vi "Lab Panel V6.00.vi"() -> ()   [LabVIEW 2017] (continued)
                      frame #2 {
                        # "switch relay off"
                        n3254 = local read "USB OUT 0"() -> (w5922:bool[])
                        n3255 = local read "USB OUT 2"() -> (w5924:bool[])
                        n3256 = local read "USB OUT 1"() -> (w5923:bool[])
                        n3257 = Insert Into Array(array=w5924, index=7, new element=FALSE) -> (w5925:bool[])
                        n3258 = call "sub vi - Drive Relays All v6.vi"("Array #2"=w5925, "Array #1"=w5923, "Array #0"=w5922) -> ()  [unwired: 8 in, 1 out]
                      }
                      frame #3 {
                        # "time delay"
                        n3259 = Wait (ms)(milliseconds to wait=300) -> ()  [unwired: 1 out]
                      }
                      frame #4 {
                        # "read all valid temp circuits"
                        n3260 = local read "LAB01-TP"() -> (w5936:bool)
                        n3261 = local read "LAB03-TP"() -> (w5934:bool)
                        n3262 = local read "LAB02-TP"() -> (w5935:bool)
                        n3263 = local read "LAB04-TP"() -> (w5933:bool)
                        n3264 = local read "LAB05-TP"() -> (w5937:bool)
                        n3265 = call "sub vi - GET ALL TEMP v7.vi"("LA01-EN"=w5936, "LA02-EN"=w5935, "LA03-EN"=w5934, "LA04-EN"=w5933, "LA05-EN"=w5937, "simulate"=w5943, "Gen Cal Value"=w5944) -> ("LOOP TIME"=→"Read Time":dbl, "Fault Counters"=→"Fault Counters":u64[], "error 1"=→"Error Temp":bool, "LA01 TEMP"=w5942:T28, "LA02 TEMP"=w5941:T28, "LA04 TEMP"=w5939:T28, "LA03 TEMP"=w5940:T28, "Errors"=→"TempErrors":bool[], "LA05 TEMP"=w5938:T28)  [unwired: 3 in, 1 out]
                        n3266 = local write "LAB01 TEMP"(w5942) -> ()
                        n3267 = local write "LAB02 TEMP"(w5941) -> ()
                        n3268 = local write "LAB03 TEMP"(w5940) -> ()
                        n3269 = local write "LAB04 TEMP"(w5939) -> ()
                        n3270 = local write "LAB05 TEMP"(w5938) -> ()
                      }
                    }
                  }
                }
              }
              frame #2 {
                n3271 = case shown="True" w5945 {
                  tunnel: w5958 -> [_ w5971]
                  tunnel: w5957 -> [_ w5970]
                  tunnel: w5956 -> [_ w5969]
                  tunnel: w5955 -> [_ w5968]
                  tunnel: w5954 -> [_ w5967]
                  tunnel: w5953 -> [_ w5966]
                  tunnel: w5952 -> [_ w5965]
                  tunnel: w5951 -> [_ w5964]
                  tunnel: w5950 -> [_ w5963]
                  tunnel: w5949 -> [_ w5962]
                  tunnel: w5948 -> [_ w5961]
                  tunnel: w5947 -> [_ w5960]
                  tunnel: w5946 -> [_ w5959]
                  frame False {
                  }
                  frame True {
                    n3272 = stacked-sequence {
                      tunnel: w5971 -> [_ w5984 w6029 w6074 w6119 w6164 _]
                      tunnel: w5970 -> [_ w5983 w6028 w6073 w6118 w6163 _]
                      tunnel: w5969 -> [_ w5973 _ _ _ _ _]
                      tunnel: w5968 -> [_ w5978 w6027 w6072 w6117 w6162 _]
                      tunnel: w5967 -> [_ w5972 _ _ _ _ _]
                      tunnel: w5966 -> [_ _ w6018 _ _ _ _]
                      tunnel: w5965 -> [_ _ w6017 _ _ _ _]
                      tunnel: w5964 -> [_ _ _ w6063 _ _ _]
                      tunnel: w5963 -> [_ _ _ w6062 _ _ _]
                      tunnel: w5962 -> [_ _ _ _ w6108 _ _]
                      tunnel: w5961 -> [_ _ _ _ w6107 _ _]
                      tunnel: w5960 -> [_ _ _ _ _ w6153 _]
                      tunnel: w5959 -> [_ _ _ _ _ w6152 _]
                      frame #0 {
                      }
                      frame #1 {
                        n3273 = case shown="False" w5984 {
                          tunnel: [w6015 w6016] -> w6000
                          tunnel: w5983 -> [_ w6016]
                          frame False {
                            n3274 = local read "CAL LAB01"() -> (w6015:T15)
                          }
                          frame True {
                          }
                        }
                        n3275 = local read "TEMP LA01"() -> (w5991:T10)
                        n3276 = local read "LAB01 TEMP"() -> (w5990:T13)
                        n3277 = call "sub vi - temperature delay v4.vi"("2-run"=w5972, "1-run"=w5973, "temp values IN"=w5991, "temp signals"=w5990) -> ("T2-N"=w5986:dbl, "T2-L"=w5987:dbl, "T1-N"=w5988:dbl, "T1-L"=w5989:dbl, "temp values OUT"=w5985:T48)  [unwired: 3 in]
                        n3278 = Unbundle By Name(w6000) -> ("1 (TL) cal"=w5995:dbl, "1 (TN) cal"=w5994:dbl, "2 (TL) cal"=w5993:dbl, "2 (TN) cal"=w5992:dbl)  [unwired: 6 out]
                        n3279 = local write "TEMP LA01"(w5985) -> ()
                        n3280 = Multiply(x=w5989, y=w5995) -> (x*y=w5982:dbl)
                        n3281 = Multiply(x=w5988, y=w5994) -> (x*y=w5980:dbl)
                        n3282 = Multiply(x=w5987, y=w5993) -> (x*y=w5977:dbl)
                        n3283 = Multiply(x=w5986, y=w5992) -> (x*y=w5976:dbl)
                        n3284 = case shown="True" w5973 {
                          tunnel: w5982 -> [w6009 w6014]
                          tunnel: w5978 -> [_ w6012]
                          tunnel: [w6009 w6013] -> w5981
                          tunnel: w5980 -> [w6008 w6011]
                          tunnel: [w6008 w6010] -> w5979
                          frame False {
                          }
                          frame True {
                            n3285 = Multiply(x=w6012, y=w6011) -> (x*y=w6010:dbl)
                            n3286 = Multiply(x=w6012, y=w6014) -> (x*y=w6013:dbl)
                          }
                        }
                        n3287 = case shown="True" w5972 {
                          tunnel: w5977 -> [w6002 w6007]
                          tunnel: w5978 -> [_ w6005]
                          tunnel: [w6002 w6006] -> w5975
                          tunnel: w5976 -> [w6001 w6004]
                          tunnel: [w6001 w6003] -> w5974
                          frame False {
                          }
                          frame True {
                            n3288 = Multiply(x=w6005, y=w6004) -> (x*y=w6003:dbl)
                            n3289 = Multiply(x=w6005, y=w6007) -> (x*y=w6006:dbl)
                          }
                        }
                        n3290 = local read "SIG LAB01-2"() -> (w5997:T2)
                        n3291 = local read "SIG LAB01-1"() -> (w5999:T2)
                        n3292 = Bundle By Name(cluster=w5999, "Tmp Live"=w5981, "Tmp Neut"=w5979) -> (w5998:T2)
                        n3293 = Bundle By Name(cluster=w5997, "Tmp Live"=w5975, "Tmp Neut"=w5974) -> (w5996:T2)
                        n3294 = local write "SIG LAB01-1"(w5998) -> ()
                        n3295 = local write "SIG LAB01-2"(w5996) -> ()
                      }
                      frame #2 {
                        n3296 = case shown="True" w6029 {
                          tunnel: [w6060 w6061] -> w6045
                          tunnel: w6028 -> [_ w6061]
                          frame False {
                            n3297 = local read "CAL LAB02"() -> (w6060:T16)
                          }
                          frame True {
                          }
                        }
                        n3298 = local read "LAB02 TEMP"() -> (w6036:T13)
                        n3299 = local read "TEMP LA02"() -> (w6035:T10)
                        n3300 = call "sub vi - temperature delay v4.vi"("2-run"=w6017, "1-run"=w6018, "temp values IN"=w6035, "temp signals"=w6036) -> ("T2-N"=w6030:dbl, "T2-L"=w6031:dbl, "T1-N"=w6032:dbl, "T1-L"=w6033:dbl, "temp values OUT"=w6034:T48)  [unwired: 3 in]
                        n3301 = Unbundle By Name(w6045) -> ("1 (TL) cal"=w6040:dbl, "1 (TN) cal"=w6039:dbl, "2 (TL) cal"=w6038:dbl, "2 (TN) cal"=w6037:dbl)  [unwired: 6 out]
                        n3302 = local write "TEMP LA02"(w6034) -> ()
                        n3303 = Multiply(x=w6033, y=w6040) -> (x*y=w6026:dbl)
                        n3304 = Multiply(x=w6032, y=w6039) -> (x*y=w6025:dbl)
                        n3305 = Multiply(x=w6031, y=w6038) -> (x*y=w6022:dbl)
                        n3306 = Multiply(x=w6030, y=w6037) -> (x*y=w6021:dbl)
                        n3307 = case shown="True" w6018 {
                          tunnel: w6026 -> [w6054 w6059]
                          tunnel: w6027 -> [_ w6057]
                          tunnel: [w6054 w6058] -> w6024
                          tunnel: w6025 -> [w6053 w6056]
                          tunnel: [w6053 w6055] -> w6023
                          frame False {
                          }
                          frame True {
                            n3308 = Multiply(x=w6057, y=w6056) -> (x*y=w6055:dbl)
                            n3309 = Multiply(x=w6057, y=w6059) -> (x*y=w6058:dbl)
                          }
                        }
                        n3310 = case shown="True" w6017 {
                          tunnel: w6022 -> [w6047 w6052]
                          tunnel: w6027 -> [_ w6050]
                          tunnel: [w6047 w6051] -> w6020
                          tunnel: w6021 -> [w6046 w6049]
                          tunnel: [w6046 w6048] -> w6019
                          frame False {
                          }
                          frame True {
                            n3311 = Multiply(x=w6050, y=w6049) -> (x*y=w6048:dbl)
                            n3312 = Multiply(x=w6050, y=w6052) -> (x*y=w6051:dbl)
                          }
                        }
                        n3313 = local read "SIG LAB02-2"() -> (w6042:T2)
                        n3314 = local read "SIG LAB02-1"() -> (w6044:T2)
                        n3315 = Bundle By Name(cluster=w6042, "Tmp Live"=w6020, "Tmp Neut"=w6019) -> (w6041:T2)
                        n3316 = Bundle By Name(cluster=w6044, "Tmp Live"=w6024, "Tmp Neut"=w6023) -> (w6043:T2)
                        n3317 = local write "SIG LAB02-1"(w6043) -> ()
                        n3318 = local write "SIG LAB02-2"(w6041) -> ()
                      }
                      frame #3 {
                        n3319 = case shown="False" w6074 {
                          tunnel: [w6105 w6106] -> w6090
                          tunnel: w6073 -> [_ w6106]
                          frame False {
                            n3320 = local read "CAL LAB03"() -> (w6105:T15)
                          }
                          frame True {
                          }
                        }
                        n3321 = local read "TEMP LA03"() -> (w6080:T10)
                        n3322 = local read "LAB03 TEMP"() -> (w6081:T13)
                        n3323 = call "sub vi - temperature delay v4.vi"("2-run"=w6062, "1-run"=w6063, "temp values IN"=w6080, "temp signals"=w6081) -> ("T2-N"=w6075:dbl, "T2-L"=w6076:dbl, "T1-N"=w6077:dbl, "T1-L"=w6078:dbl, "temp values OUT"=w6079:T48)  [unwired: 3 in]
                        n3324 = Unbundle By Name(w6090) -> ("1 (TL) cal"=w6085:dbl, "1 (TN) cal"=w6084:dbl, "2 (TL) cal"=w6083:dbl, "2 (TN) cal"=w6082:dbl)  [unwired: 6 out]
                        n3325 = local write "TEMP LA03"(w6079) -> ()
                        n3326 = Multiply(x=w6078, y=w6085) -> (x*y=w6071:dbl)
                        n3327 = Multiply(x=w6077, y=w6084) -> (x*y=w6070:dbl)
                        n3328 = Multiply(x=w6076, y=w6083) -> (x*y=w6067:dbl)
                        n3329 = Multiply(x=w6075, y=w6082) -> (x*y=w6066:dbl)
                        n3330 = case shown="True" w6062 {
                          tunnel: w6067 -> [w6092 w6097]
                          tunnel: w6072 -> [_ w6095]
                          tunnel: [w6092 w6096] -> w6065
                          tunnel: w6066 -> [w6091 w6094]
                          tunnel: [w6091 w6093] -> w6064
                          frame False {
                          }
                          frame True {
                            n3331 = Multiply(x=w6095, y=w6094) -> (x*y=w6093:dbl)
                            n3332 = Multiply(x=w6095, y=w6097) -> (x*y=w6096:dbl)
                          }
                        }
                        n3333 = case shown="True" w6063 {
                          tunnel: w6071 -> [w6099 w6104]
                          tunnel: w6072 -> [_ w6102]
                          tunnel: [w6099 w6103] -> w6069
                          tunnel: w6070 -> [w6098 w6101]
                          tunnel: [w6098 w6100] -> w6068
                          frame False {
                          }
                          frame True {
                            n3334 = Multiply(x=w6102, y=w6101) -> (x*y=w6100:dbl)
                            n3335 = Multiply(x=w6102, y=w6104) -> (x*y=w6103:dbl)
                          }
                        }
                        n3336 = local read "SIG LAB03-2"() -> (w6087:T2)
                        n3337 = local read "SIG LAB03-1"() -> (w6089:T2)
                        n3338 = Bundle By Name(cluster=w6087, "Tmp Live"=w6065, "Tmp Neut"=w6064) -> (w6086:T2)
                        n3339 = Bundle By Name(cluster=w6089, "Tmp Live"=w6069, "Tmp Neut"=w6068) -> (w6088:T2)
                        n3340 = local write "SIG LAB03-2"(w6086) -> ()
                        n3341 = local write "SIG LAB03-1"(w6088) -> ()
                      }
                      frame #4 {
                        n3342 = case shown="False" w6119 {
                          tunnel: [w6150 w6151] -> w6135
                          tunnel: w6118 -> [_ w6151]
                          frame False {
                            n3343 = local read "CAL LAB04"() -> (w6150:T15)
                          }
                          frame True {
                          }
                        }
                        n3344 = local read "LAB04 TEMP"() -> (w6125:T13)
                        n3345 = local read "TEMP LA04"() -> (w6126:T10)
                        n3346 = call "sub vi - temperature delay v4.vi"("2-run"=w6107, "1-run"=w6108, "temp values IN"=w6126, "temp signals"=w6125) -> ("T2-N"=w6120:dbl, "T2-L"=w6121:dbl, "T1-N"=w6122:dbl, "T1-L"=w6123:dbl, "temp values OUT"=w6124:T48)  [unwired: 3 in]
                        n3347 = Unbundle By Name(w6135) -> ("1 (TL) cal"=w6130:dbl, "1 (TN) cal"=w6129:dbl, "2 (TL) cal"=w6128:dbl, "2 (TN) cal"=w6127:dbl)  [unwired: 6 out]
                        n3348 = local write "TEMP LA04"(w6124) -> ()
                        n3349 = Multiply(x=w6123, y=w6130) -> (x*y=w6116:dbl)
                        n3350 = Multiply(x=w6122, y=w6129) -> (x*y=w6115:dbl)
                        n3351 = Multiply(x=w6121, y=w6128) -> (x*y=w6112:dbl)
                        n3352 = Multiply(x=w6120, y=w6127) -> (x*y=w6111:dbl)
                        n3353 = case shown="True" w6107 {
                          tunnel: w6112 -> [w6137 w6142]
                          tunnel: w6117 -> [_ w6140]
                          tunnel: [w6137 w6141] -> w6110
                          tunnel: w6111 -> [w6136 w6139]
                          tunnel: [w6136 w6138] -> w6109
                          frame False {
                          }
                          frame True {
                            n3354 = Multiply(x=w6140, y=w6139) -> (x*y=w6138:dbl)
                            n3355 = Multiply(x=w6140, y=w6142) -> (x*y=w6141:dbl)
                          }
                        }
                        n3356 = case shown="True" w6108 {
                          tunnel: w6116 -> [w6144 w6149]
                          tunnel: w6117 -> [_ w6147]
                          tunnel: [w6144 w6148] -> w6114
                          tunnel: w6115 -> [w6143 w6146]
                          tunnel: [w6143 w6145] -> w6113
                          frame False {
                          }
                          frame True {
                            n3357 = Multiply(x=w6147, y=w6146) -> (x*y=w6145:dbl)
                            n3358 = Multiply(x=w6147, y=w6149) -> (x*y=w6148:dbl)
                          }
                        }
                        n3359 = local read "SIG LAB04-2"() -> (w6132:T2)
                        n3360 = local read "SIG LAB04-1"() -> (w6134:T2)
                        n3361 = Bundle By Name(cluster=w6132, "Tmp Live"=w6110, "Tmp Neut"=w6109) -> (w6131:T2)
                        n3362 = Bundle By Name(cluster=w6134, "Tmp Live"=w6114, "Tmp Neut"=w6113) -> (w6133:T2)
                        n3363 = local write "SIG LAB04-2"(w6131) -> ()
                        n3364 = local write "SIG LAB04-1"(w6133) -> ()
                      }
                      frame #5 {
                        n3365 = case shown="False" w6164 {
                          tunnel: [w6195 w6196] -> w6180
                          tunnel: w6163 -> [_ w6196]
                          frame False {
                            n3366 = local read "CAL LAB05"() -> (w6195:T15)
                          }
                          frame True {
                          }
                        }
                        n3367 = local read "LAB05 TEMP"() -> (w6170:T13)
                        n3368 = local read "TEMP LA05"() -> (w6171:T10)
                        n3369 = call "sub vi - temperature delay v4.vi"("2-run"=w6152, "1-run"=w6153, "temp values IN"=w6171, "temp signals"=w6170) -> ("T2-N"=w6166:dbl, "T2-L"=w6167:dbl, "T1-N"=w6168:dbl, "T1-L"=w6169:dbl, "temp values OUT"=w6165:T48)  [unwired: 3 in]
                        n3370 = local write "TEMP LA05"(w6165) -> ()
                        n3371 = Unbundle By Name(w6180) -> ("1 (TL) cal"=w6172:dbl, "1 (TN) cal"=w6175:dbl, "2 (TL) cal"=w6174:dbl, "2 (TN) cal"=w6173:dbl)  [unwired: 6 out]
                        n3372 = Multiply(x=w6169, y=w6172) -> (x*y=w6161:dbl)
                        n3373 = Multiply(x=w6168, y=w6175) -> (x*y=w6160:dbl)
                        n3374 = Multiply(x=w6167, y=w6174) -> (x*y=w6157:dbl)
                        n3375 = Multiply(x=w6166, y=w6173) -> (x*y=w6156:dbl)
                        n3376 = case shown="True" w6152 {
                          tunnel: w6157 -> [w6182 w6187]
                          tunnel: w6162 -> [_ w6185]
                          tunnel: [w6182 w6186] -> w6155
                          tunnel: w6156 -> [w6181 w6184]
                          tunnel: [w6181 w6183] -> w6154
                          frame False {
                          }
                          frame True {
                            n3377 = Multiply(x=w6185, y=w6184) -> (x*y=w6183:dbl)
                            n3378 = Multiply(x=w6185, y=w6187) -> (x*y=w6186:dbl)
                          }
                        }
                        n3379 = case shown="True" w6153 {
                          tunnel: w6161 -> [w6189 w6194]
                          tunnel: w6162 -> [_ w6192]
                          tunnel: [w6189 w6193] -> w6159
                          tunnel: w6160 -> [w6188 w6191]
                          tunnel: [w6188 w6190] -> w6158
                          frame False {
                          }
                          frame True {
                            n3380 = Multiply(x=w6192, y=w6191) -> (x*y=w6190:dbl)
                            n3381 = Multiply(x=w6192, y=w6194) -> (x*y=w6193:dbl)
                          }
                        }
                        n3382 = local read "SIG LAB05-1"() -> (w6179:T2)
                        n3383 = Bundle By Name(cluster=w6179, "Tmp Live"=w6159, "Tmp Neut"=w6158) -> (w6178:T2)
                        n3384 = local read "SIG LAB05-2"() -> (w6177:T2)
                        n3385 = Bundle By Name(cluster=w6177, "Tmp Live"=w6155, "Tmp Neut"=w6154) -> (w6176:T2)
                        n3386 = local write "SIG LAB05-1"(w6178) -> ()
                        n3387 = local write "SIG LAB05-2"(w6176) -> ()
                      }
                      frame #6 {
                        w6297 = 150.0
                        # "check for thermocouple error, output >150 deg??"
                        n3388 = local read "SIG LAB01-2"() -> (w6306:T2)
                        n3389 = local read "SIG LAB01-1"() -> (w6307:T2)
                        n3390 = local read "SIG LAB04-1"() -> (w6300:T2)
                        n3391 = local read "SIG LAB04-2"() -> (w6301:T2)
                        n3392 = Unbundle By Name(w6307) -> ("Tmp Live"=w6235:dbl, "Tmp Neut"=w6233:dbl)
                        n3393 = Unbundle(w6301) -> ("Tmp Live"=w6211:dbl, "Tmp Neut"=w6210:dbl)  [unwired: 3 out]
                        n3394 = Unbundle(w6306) -> ("Tmp Live"=w6232:dbl, "Tmp Neut"=w6230:dbl)  [unwired: 3 out]
                        n3395 = Unbundle(w6300) -> ("Tmp Live"=w6212:dbl, "Tmp Neut"=w6205:dbl)  [unwired: 3 out]
                        n3396 = Absolute Value(x=w6212) -> (abs(x)=w6206:dbl)
                        n3397 = Absolute Value(x=w6205) -> (abs(x)=w6207:dbl)
                        n3398 = Absolute Value(x=w6211) -> (abs(x)=w6209:dbl)
                        n3399 = Absolute Value(x=w6210) -> (abs(x)=w6208:dbl)
                        n3400 = Absolute Value(x=w6232) -> (abs(x)=w6231:dbl)
                        n3401 = Absolute Value(x=w6230) -> (abs(x)=w6229:dbl)
                        n3402 = Absolute Value(x=w6233) -> (abs(x)=w6234:dbl)
                        n3403 = Absolute Value(x=w6235) -> (abs(x)=w6236:dbl)
                        n3404 = Greater?(x=w6208, y=w6297) -> (0:w6273:bool)
                        "LA04-2 (TN)" <- w6273
                        n3405 = Greater?(x=w6229, y=w6297) -> (0:w6285:bool)
                        "LA01-2 (TN)" <- w6285
                        n3406 = Greater?(x=w6209, y=w6297) -> (0:w6274:bool)
                        "LA04-2 (TL)" <- w6274
                        n3407 = Greater?(x=w6231, y=w6297) -> (0:w6286:bool)
                        "LA01-2 (TL)" <- w6286
                        n3408 = Greater?(x=w6207, y=w6297) -> (0:w6275:bool)
                        "LA04-1 (TN)" <- w6275
                        n3409 = Greater?(x=w6234, y=w6297) -> (0:w6296:bool)
                        "LA01-1 (TN)" <- w6296
                        n3410 = Greater?(x=w6206, y=w6297) -> (0:w6276:bool)
                        "LA04-1 (TL)" <- w6276
                        n3411 = Greater?(x=w6236, y=w6297) -> (0:w6295:bool)
                        "LA01-1 (TL)" <- w6295
                        n3412 = Or(x=w6296, y=w6295) -> (x .or. y?=w6294:bool)
                        n3413 = Or(x=w6273, y=w6274) -> (x .or. y?=w6284:bool)
                        n3414 = Or(x=w6286, y=w6285) -> (x .or. y?=w6290:bool)
                        n3415 = Or(x=w6275, y=w6276) -> (x .or. y?=w6280:bool)
                        n3416 = Select(t=u32 16711680, s=w6294, f=u32 13816530) -> (s? t:f=w6291:u32)
                        n3417 = Select(t=u32 16711680, s=w6284, f=u32 13816530) -> (s? t:f=w6281:u32)
                        n3418 = Select(t=u32 16711680, s=w6290, f=u32 13816530) -> (s? t:f=w6287:u32)
                        n3419 = Select(t=u32 16711680, s=w6280, f=u32 13816530) -> (s? t:f=w6277:u32)
                        n3420 = property on="SIG LAB01-1" class="Clust (strict)"("Color"=w6291) -> ()  [unwired: 2 in, 2 out]
                        n3421 = property on="SIG LAB01-2" class="Clust (strict)"("Color"=w6287) -> ()  [unwired: 2 in, 2 out]
                        n3422 = property on="SIG LAB04-2" class="Clust (strict)"("Color"=w6281) -> ()  [unwired: 2 in, 2 out]
                        n3423 = property on="SIG LAB04-1" class="Clust (strict)"("Color"=w6277) -> ()  [unwired: 2 in, 2 out]
                        n3424 = local read "SIG LAB02-1"() -> (w6304:T2)
                        n3425 = local read "SIG LAB02-2"() -> (w6305:T2)
                        n3426 = local read "SIG LAB05-2"() -> (w6298:T2)
                        n3427 = local read "SIG LAB05-1"() -> (w6299:T2)
                        n3428 = Unbundle(w6305) -> ("Tmp Live"=w6224:dbl, "Tmp Neut"=w6222:dbl)  [unwired: 3 out]
                        n3429 = Unbundle(w6304) -> ("Tmp Live"=w6228:dbl, "Tmp Neut"=w6227:dbl)  [unwired: 3 out]
                        n3430 = Unbundle(w6298) -> ("Tmp Live"=w6200:dbl, "Tmp Neut"=w6198:dbl)  [unwired: 3 out]
                        n3431 = Unbundle(w6299) -> ("Tmp Live"=w6204:dbl, "Tmp Neut"=w6202:dbl)  [unwired: 3 out]
                        n3432 = Absolute Value(x=w6224) -> (abs(x)=w6223:dbl)
                        n3433 = Absolute Value(x=w6222) -> (abs(x)=w6221:dbl)
                        n3434 = Absolute Value(x=w6227) -> (abs(x)=w6225:dbl)
                        n3435 = Absolute Value(x=w6228) -> (abs(x)=w6226:dbl)
                        n3436 = Absolute Value(x=w6200) -> (abs(x)=w6199:dbl)
                        n3437 = Absolute Value(x=w6198) -> (abs(x)=w6197:dbl)
                        n3438 = Absolute Value(x=w6204) -> (abs(x)=w6203:dbl)
                        n3439 = Absolute Value(x=w6202) -> (abs(x)=w6201:dbl)
                        n3440 = Greater?(x=w6221, y=w6297) -> (0:w6249:bool)
                        "LA02-2 (TN)" <- w6249
                        n3441 = Greater?(x=w6223, y=w6297) -> (0:w6250:bool)
                        "LA02-2 (TL)" <- w6250
                        n3442 = Greater?(x=w6225, y=w6297) -> (0:w6252:bool)
                        "LA02-1 (TN)" <- w6252
                        n3443 = Greater?(x=w6226, y=w6297) -> (0:w6251:bool)
                        "LA02-1 (TL)" <- w6251
                        n3444 = Greater?(x=w6197, y=w6297) -> (0:w6261:bool)
                        "LA05-2 (TN)" <- w6261
                        n3445 = Greater?(x=w6199, y=w6297) -> (0:w6262:bool)
                        "LA05-2 (TL)" <- w6262
                        n3446 = Greater?(x=w6201, y=w6297) -> (0:w6263:bool)
                        "LA05-1 (TN)" <- w6263
                        n3447 = Greater?(x=w6203, y=w6297) -> (0:w6264:bool)
                        "LA05-1 (TL)" <- w6264
                        n3448 = Or(x=w6252, y=w6251) -> (x .or. y?=w6260:bool)
                        n3449 = Or(x=w6250, y=w6249) -> (x .or. y?=w6256:bool)
                        n3450 = Or(x=w6264, y=w6263) -> (x .or. y?=w6272:bool)
                        n3451 = Or(x=w6262, y=w6261) -> (x .or. y?=w6268:bool)
                        n3452 = Select(t=u32 16711680, s=w6260, f=u32 13816530) -> (s? t:f=w6257:u32)
                        n3453 = Select(t=u32 16711680, s=w6256, f=u32 13816530) -> (s? t:f=w6253:u32)
                        n3454 = Select(t=u32 16711680, s=w6272, f=u32 13816530) -> (s? t:f=w6269:u32)
                        n3455 = local read "SIG LAB03-1"() -> (w6302:T2)
                        n3456 = Select(t=u32 16711680, s=w6268, f=u32 13816530) -> (s? t:f=w6265:u32)
                        n3457 = property on="SIG LAB02-1" class="Clust (strict)"("Color"=w6257) -> ()  [unwired: 2 in, 2 out]
                        n3458 = property on="SIG LAB02-2" class="Clust (strict)"("Color"=w6253) -> ()  [unwired: 2 in, 2 out]
                        n3459 = local read "SIG LAB03-2"() -> (w6303:T2)
                        n3460 = property on="SIG LAB05-1" class="Clust (strict)"("Color"=w6269) -> ()  [unwired: 2 in, 2 out]
                        n3461 = property on="SIG LAB05-2" class="Clust (strict)"("Color"=w6265) -> ()  [unwired: 2 in, 2 out]
                        n3462 = Unbundle(w6303) -> ("Tmp Live"=w6216:dbl, "Tmp Neut"=w6214:dbl)  [unwired: 3 out]
                        n3463 = Unbundle(w6302) -> ("Tmp Live"=w6220:dbl, "Tmp Neut"=w6218:dbl)  [unwired: 3 out]
                        n3464 = Absolute Value(x=w6216) -> (abs(x)=w6215:dbl)
                        n3465 = Absolute Value(x=w6214) -> (abs(x)=w6213:dbl)
                        n3466 = Absolute Value(x=w6220) -> (abs(x)=w6219:dbl)
                        n3467 = Absolute Value(x=w6218) -> (abs(x)=w6217:dbl)
                        n3468 = Greater?(x=w6213, y=w6297) -> (0:w6237:bool)
                        "LA03-2 (TN)" <- w6237
                        n3469 = Greater?(x=w6215, y=w6297) -> (0:w6238:bool)
                        "LA03-2 (TL)" <- w6238
                        n3470 = Greater?(x=w6217, y=w6297) -> (0:w6240:bool)
                        "LA03-1 (TN)" <- w6240
                        n3471 = Greater?(x=w6219, y=w6297) -> (0:w6239:bool)
                        "LA03-1 (TL)" <- w6239
                        n3472 = Or(x=w6240, y=w6239) -> (x .or. y?=w6248:bool)
                        n3473 = Or(x=w6238, y=w6237) -> (x .or. y?=w6244:bool)
                        n3474 = Select(t=u32 16711680, s=w6248, f=u32 13816530) -> (s? t:f=w6245:u32)
                        n3475 = Select(t=u32 16711680, s=w6244, f=u32 13816530) -> (s? t:f=w6241:u32)
                        n3476 = property on="SIG LAB03-1" class="Clust (strict)"("Color"=w6245) -> ()  [unwired: 2 in, 2 out]
                        n3477 = property on="SIG LAB03-2" class="Clust (strict)"("Color"=w6241) -> ()  [unwired: 2 in, 2 out]
                      }
                    }
                  }
                }
              }
            }
          }
          frame #22 {
            # "SAVE ON AMPS VALUES FOR REPORT FILE"
            # "write data to display panel"
            n3478 = global write "Global display 1.vi" "TEST 5-2"(w6343) -> ()
            n3479 = global write "Global display 1.vi" "TEST 4-2"(w6345) -> ()
            n3480 = global write "Global display 1.vi" "TEST 1-2"(w6351) -> ()
            n3481 = global write "Global display 1.vi" "TEST 3-1"(w6348) -> ()
            n3482 = global write "Global display 1.vi" "TEST 5-1"(w6344) -> ()
            n3483 = global write "Global display 1.vi" "TEST 1-1"(w6352) -> ()
            n3484 = global write "Global display 1.vi" "TEST 3-2"(w6347) -> ()
            n3485 = global write "Global display 1.vi" "TEST 4-1"(w6346) -> ()
            n3486 = global write "Global display 1.vi" "TEST 2-2"(w6349) -> ()
            n3487 = global write "Global display 1.vi" "TEST 2-1"(w6350) -> ()
            n3488 = global read "Global display 3.vi" "log 1-1"() -> (→"LOG LAB01-1":string)
            n3489 = global read "Global display 3.vi" "log 3-1"() -> (→"LOG LAB03-1":string)
            n3490 = global read "Global display 3.vi" "log 1-2"() -> (→"LOG LAB01-2":string)
            n3491 = property on="Tab Control 2" class="TabCtl (strict)"() -> ("Pages"=w6342:refnum<vi>[])  [unwired: 2 in, 2 out]
            n3492 = global read "Global display 3.vi" "log 2-1"() -> (→"LOG LAB02-1":string)
            n3493 = global read "Global display 3.vi" "log 2-2"() -> (→"LOG LAB02-2":string)
            n3494 = global read "Global display 3.vi" "log 4-2"() -> (→"LOG LAB04-2":string)
            n3495 = global read "Global display 3.vi" "log 5-2"() -> (→"LOG LAB05-2":string)
            n3496 = global read "Global display 3.vi" "log 5-1"() -> (→"LOG LAB05-1":string)
            n3497 = global read "Global display 3.vi" "log 4-1"() -> (→"LOG LAB04-1":string)
            n3498 = global read "Global display 3.vi" "log 3-2"() -> (→"LOG LAB03-2":string)
            n3499 = Index Array(array=w6342, index=8) -> (element=w6340:refnum<vi>)
            n3500 = property class="Page"(reference=w6340) -> ("PageVis"=w6339:bool)  [unwired: 1 in, 2 out]
            n3501 = local read "DISP LAB03-1"() -> (w6378:T4)
            n3502 = local read "DISP LAB04-2"() -> (w6375:T4)
            n3503 = local read "DISP LAB05-1"() -> (w6374:T4)
            n3504 = local read "DISP LAB01-2"() -> (w6381:T4)
            n3505 = local read "DISP LAB02-1"() -> (w6380:T4)
            n3506 = local read "DISP LAB02-2"() -> (w6379:T4)
            n3507 = local read "DISP LAB04-1"() -> (w6376:T4)
            n3508 = local read "DISP LAB05-2"() -> (w6373:T4)
            n3509 = local read "DISP LAB01-1"() -> (w6382:T4)
            n3510 = local read "DISP LAB03-2"() -> (w6377:T4)
            n3511 = global write "Global display 3.vi" "admin"(w6339) -> ()
            n3512 = local read "O/I  LAB05-2"() -> (w6393:bool)
            n3513 = local read "O/I  LAB05-1"() -> (w6394:bool)
            n3514 = local read "O/I  LAB03-2"() -> (w6397:bool)
            n3515 = local read "O/I  LAB04-2"() -> (w6395:bool)
            n3516 = local read "O/I  LAB04-1"() -> (w6396:bool)
            n3517 = local read "O/I  LAB03-1"() -> (w6398:bool)
            n3518 = local read "O/I  LAB01-2"() -> (w6401:bool)
            n3519 = local read "O/I  LAB01-1"() -> (w6402:bool)
            n3520 = local read "O/I  LAB02-1"() -> (w6400:bool)
            n3521 = local read "O/I  LAB02-2"() -> (w6399:bool)
            n3522 = global write "Global display 1.vi" "5-2 O/F"(w6393) -> ()
            n3523 = global write "Global display 1.vi" "5-1 O/F"(w6394) -> ()
            n3524 = global write "Global display 1.vi" "4-1 O/F"(w6396) -> ()
            n3525 = global write "Global display 1.vi" "4-2 O/F"(w6395) -> ()
            n3526 = global write "Global display 2.vi" "DISP LAB02-1"(w6380) -> ()
            n3527 = global write "Global display 2.vi" "DISP LAB02-2"(w6379) -> ()
            n3528 = global write "Global display 2.vi" "DISP LAB05-1"(w6374) -> ()
            n3529 = global write "Global display 2.vi" "DISP LAB05-2"(w6373) -> ()
            n3530 = global write "Global display 1.vi" "3-2 O/F"(w6397) -> ()
            n3531 = global write "Global display 2.vi" "DISP LAB01-2"(w6381) -> ()
            n3532 = global write "Global display 2.vi" "DISP LAB04-2"(w6375) -> ()
            n3533 = global write "Global display 2.vi" "DISP LAB01-1"(w6382) -> ()
            n3534 = global write "Global display 2.vi" "DISP LAB03-1"(w6378) -> ()
            n3535 = global write "Global display 1.vi" "3-1 O/F"(w6398) -> ()
            n3536 = global write "Global display 2.vi" "DISP LAB04-1"(w6376) -> ()
            n3537 = global write "Global display 1.vi" "2-2 O/F"(w6399) -> ()
            n3538 = global write "Global display 2.vi" "DISP LAB03-2"(w6377) -> ()
            n3539 = global write "Global display 1.vi" "2-1 O/F"(w6400) -> ()
            n3540 = global write "Global display 1.vi" "1-2 O/F"(w6401) -> ()
            n3541 = global write "Global display 1.vi" "1-1 O/F"(w6402) -> ()
            n3542 = local read "run lab05-2"() -> (w6383:bool)
            n3543 = local read "run lab04-1"() -> (w6386:bool)
            n3544 = local read "run lab04-2"() -> (w6385:bool)
            n3545 = local read "run lab05-1"() -> (w6384:bool)
            n3546 = local read "TEMP START LAB02-2"() -> (w6325:cluster{"TL":dbl, "TN":dbl})
            n3547 = local read "TEMP START LAB01-2"() -> (w6327:cluster{"TL":dbl, "TN":dbl})
            n3548 = local read "TEMP START LAB02-1"() -> (w6326:cluster{"TL":dbl, "TN":dbl})
            n3549 = local read "TEMP START LAB04-1"() -> (w6322:cluster{"TL":dbl, "TN":dbl})
            n3550 = local read "TEMP START LAB04-2"() -> (w6321:cluster{"TL":dbl, "TN":dbl})
            n3551 = local read "run lab03-2"() -> (w6387:bool)
            n3552 = local read "TEMP START LAB01-1"() -> (w6328:cluster{"TL":dbl, "TN":dbl})
            n3553 = local read "TEMP START LAB05-2"() -> (w6319:cluster{"TL":dbl, "TN":dbl})
            n3554 = local read "TEMP START LAB05-1"() -> (w6320:cluster{"TL":dbl, "TN":dbl})
            n3555 = local read "run lab02-1"() -> (w6390:bool)
            n3556 = local read "run lab03-1"() -> (w6388:bool)
            n3557 = local read "TEMP START LAB03-2"() -> (w6323:cluster{"TL":dbl, "TN":dbl})
            n3558 = local read "run lab01-2"() -> (w6391:bool)
            n3559 = local read "run lab02-2"() -> (w6389:bool)
            n3560 = local read "TEMP START LAB03-1"() -> (w6324:cluster{"TL":dbl, "TN":dbl})
            n3561 = local read "run lab01-1"() -> (w6392:bool)
            n3562 = global write "Global display 1.vi" "5-2 R/S"(w6383) -> ()
            n3563 = global write "Global display 1.vi" "5-1 R/S"(w6384) -> ()
            n3564 = global write "Global display 1.vi" "4-2 R/S"(w6385) -> ()
            n3565 = global write "Global display 1.vi" "4-1 R/S"(w6386) -> ()
            n3566 = global write "Global display 1.vi" "3-2 R/S"(w6387) -> ()
            n3567 = global write "Global display 1.vi" "1-2 R/S"(w6391) -> ()
            n3568 = global write "Global display 1.vi" "2-1 R/S"(w6390) -> ()
            n3569 = global write "Global display 1.vi" "3-1 R/S"(w6388) -> ()
            n3570 = global write "Global display 1.vi" "2-2 R/S"(w6389) -> ()
            n3571 = global write "Global display 1.vi" "1-1 R/S"(w6392) -> ()
            n3572 = local read "SET LAB05-2"() -> (w6363:T5)
            n3573 = local read "SET LAB05-1"() -> (w6364:T5)
            n3574 = local read "SET LAB04-1"() -> (w6366:T5)
            n3575 = local read "SET LAB04-2"() -> (w6365:T5)
            n3576 = local read "SET LAB01-1"() -> (w6372:T6)
            n3577 = local read "SET LAB03-1"() -> (w6368:T5)
            n3578 = local read "SET LAB03-2"() -> (w6367:T5)
            n3579 = local read "SET LAB02-2"() -> (w6369:T5)
            n3580 = local read "SET LAB01-2"() -> (w6371:T5)
            n3581 = local read "SET LAB02-1"() -> (w6370:T5)
            n3582 = global write "Global display 3.vi" "TEMP ST 05-2"(w6319) -> ()
            n3583 = global write "Global display 3.vi" "TEMP ST 05-1"(w6320) -> ()
            n3584 = global write "Global display 3.vi" "TEMP ST 03-2"(w6323) -> ()
            n3585 = global write "Global display 3.vi" "TEMP ST 04-2"(w6321) -> ()
            n3586 = global write "Global display 3.vi" "TEMP ST 01-1"(w6328) -> ()
            n3587 = global write "Global display 3.vi" "TEMP ST 01-2"(w6327) -> ()
            n3588 = global write "Global display 3.vi" "TEMP ST 04-1"(w6322) -> ()
            n3589 = global write "Global display 3.vi" "TEMP ST 02-1"(w6326) -> ()
            n3590 = global write "Global display 3.vi" "TEMP ST 02-2"(w6325) -> ()
            n3591 = global write "Global display 3.vi" "TEMP ST 03-1"(w6324) -> ()
            n3592 = global write "Global display 2.vi" "SET LAB05-2"(w6363) -> ()
            n3593 = global write "Global display 2.vi" "SET LAB05-1"(w6364) -> ()
            n3594 = global write "Global display 2.vi" "SET LAB04-1"(w6366) -> ()
            n3595 = global write "Global display 2.vi" "SET LAB01-1"(w6372) -> ()
            n3596 = global write "Global display 2.vi" "SET LAB04-2"(w6365) -> ()
            n3597 = global write "Global display 2.vi" "SET LAB03-2"(w6367) -> ()
            n3598 = global write "Global display 2.vi" "SET LAB02-2"(w6369) -> ()
            n3599 = global write "Global display 2.vi" "SET LAB03-1"(w6368) -> ()
            n3600 = global write "Global display 2.vi" "SET LAB01-2"(w6371) -> ()
            n3601 = global write "Global display 2.vi" "SET LAB02-1"(w6370) -> ()
            n3602 = local read "TEMP RISE LAB05-1"() -> (w6310:cluster{"TL":dbl, "TN":dbl})
            n3603 = local read "TEMP RISE LAB05-2"() -> (w6309:cluster{"TL":dbl, "TN":dbl})
            n3604 = local read "TEMP RISE LAB04-2"() -> (w6311:cluster{"TL":dbl, "TN":dbl})
            n3605 = local read "TEMP RISE LAB04-1"() -> (w6312:cluster{"TL":dbl, "TN":dbl})
            n3606 = local read "TEMP RISE LAB03-2"() -> (w6313:cluster{"TL":dbl, "TN":dbl})
            n3607 = local read "TEMP RISE LAB03-1"() -> (w6314:cluster{"TL":dbl, "TN":dbl})
            n3608 = local read "TEMP RISE LAB01-2"() -> (w6317:cluster{"TL":dbl, "TN":dbl})
            n3609 = local read "TEMP RISE LAB02-2"() -> (w6315:cluster{"TL":dbl, "TN":dbl})
            n3610 = local read "TEMP RISE LAB01-1"() -> (w6318:cluster{"TL":dbl, "TN":dbl})
            n3611 = local read "TEMP RISE LAB02-1"() -> (w6316:cluster{"TL":dbl, "TN":dbl})
            n3612 = local read "RESULT LAB01-1"() -> (w6362:bool)
            n3613 = local read "RESULT LAB03-2"() -> (w6357:bool)
            n3614 = local read "RESULT LAB04-1"() -> (w6356:bool)
            n3615 = local read "RESULT LAB04-2"() -> (w6355:bool)
            n3616 = local read "RESULT LAB02-2"() -> (w6359:bool)
            n3617 = local read "RESULT LAB01-2"() -> (w6361:bool)
            n3618 = local read "RESULT LAB02-1"() -> (w6360:bool)
            n3619 = local read "RESULT LAB03-1"() -> (w6358:bool)
            n3620 = local read "RESULT LAB05-1"() -> (w6354:bool)
            n3621 = local read "RESULT LAB05-2"() -> (w6353:bool)
            n3622 = local read "Amps Fail level"() -> (w6308:dbl)
            n3623 = stacked-sequence {
              tunnel: w6308 -> [w6404 w6409 w6414 w6419 w6424 w6429 w6434 w6439 w6444 w6449]
              frame #0 {
                n3624 = local read "SIG LAB01-1"() -> (w6406:T2)
                n3625 = Unbundle(w6406) -> ("AMPS"=w6405:dbl)  [unwired: 4 out]
                n3626 = Greater?(x=w6405, y=w6404) -> (0:w6403:bool)
                n3627 = case shown="True" w6403 {
                  frame False {
                  }
                  frame True {
                    n3628 = local read "ON L01-1"() -> (w6407:cluster{"amps":dbl, "volts":dbl, "pf":dbl})
                    n3629 = global write "Global display 2.vi" "ON L01-1"(w6407) -> ()
                  }
                }
              }
              frame #1 {
                n3630 = local read "SIG LAB01-2"() -> (w6411:T2)
                n3631 = Unbundle By Name(w6411) -> ("AMPS"=w6410:dbl)
                n3632 = Greater?(x=w6410, y=w6409) -> (0:w6408:bool)
                n3633 = case shown="True" w6408 {
                  frame False {
                  }
                  frame True {
                    n3634 = local read "ON L01-2"() -> (w6412:cluster{"amps":dbl, "volts":dbl, "pf":dbl})
                    n3635 = global write "Global display 2.vi" "ON L01-2"(w6412) -> ()
                  }
                }
              }
              frame #2 {
                n3636 = local read "SIG LAB02-1"() -> (w6416:T2)
                n3637 = Unbundle(w6416) -> ("AMPS"=w6415:dbl)  [unwired: 4 out]
                n3638 = Greater?(x=w6415, y=w6414) -> (0:w6413:bool)
                n3639 = case shown="True" w6413 {
                  frame False {
                  }
                  frame True {
                    n3640 = local read "ON L02-1"() -> (w6417:cluster{"amps":dbl, "volts":dbl, "pf":dbl})
                    n3641 = global write "Global display 2.vi" "ON L02-1"(w6417) -> ()
                  }
                }
              }
              frame #3 {
                n3642 = local read "SIG LAB02-2"() -> (w6421:T2)
                n3643 = Unbundle(w6421) -> ("AMPS"=w6420:dbl)  [unwired: 4 out]
                n3644 = Greater?(x=w6420, y=w6419) -> (0:w6418:bool)
                n3645 = case shown="True" w6418 {
                  frame False {
                  }
                  frame True {
                    n3646 = local read "ON L02-2"() -> (w6422:cluster{"amps":dbl, "volts":dbl, "pf":dbl})
                    n3647 = global write "Global display 2.vi" "ON L02-2"(w6422) -> ()
                  }
                }
              }
              frame #4 {
                n3648 = local read "SIG LAB03-1"() -> (w6426:T2)
                n3649 = Unbundle(w6426) -> ("AMPS"=w6425:dbl)  [unwired: 4 out]
                n3650 = Greater?(x=w6425, y=w6424) -> (0:w6423:bool)
                n3651 = case shown="True" w6423 {
                  frame False {
                  }
                  frame True {
                    n3652 = local read "ON L03-1"() -> (w6427:cluster{"amps":dbl, "volts":dbl, "pf":dbl})
                    n3653 = global write "Global display 2.vi" "ON L03-1"(w6427) -> ()
                  }
                }
              }
              frame #5 {
                n3654 = local read "SIG LAB03-2"() -> (w6431:T2)
                n3655 = Unbundle(w6431) -> ("AMPS"=w6430:dbl)  [unwired: 4 out]
                n3656 = Greater?(x=w6430, y=w6429) -> (0:w6428:bool)
                n3657 = case shown="True" w6428 {
                  frame False {
                  }
                  frame True {
                    n3658 = local read "ON L03-2"() -> (w6432:cluster{"amps":dbl, "volts":dbl, "pf":dbl})
                    n3659 = global write "Global display 2.vi" "ON L03-2"(w6432) -> ()
                  }
                }
              }
              frame #6 {
                n3660 = local read "SIG LAB04-1"() -> (w6436:T2)
                n3661 = Unbundle(w6436) -> ("AMPS"=w6435:dbl)  [unwired: 4 out]
                n3662 = Greater?(x=w6435, y=w6434) -> (0:w6433:bool)
                n3663 = case shown="True" w6433 {
                  frame False {
                  }
                  frame True {
                    n3664 = local read "ON L04-1"() -> (w6437:cluster{"amps":dbl, "volts":dbl, "pf":dbl})
                    n3665 = global write "Global display 2.vi" "ON L04-1"(w6437) -> ()
                  }
                }
              }
              frame #7 {
                n3666 = local read "SIG LAB04-2"() -> (w6441:T2)
                n3667 = Unbundle(w6441) -> ("AMPS"=w6440:dbl)  [unwired: 4 out]
                n3668 = Greater?(x=w6440, y=w6439) -> (0:w6438:bool)
                n3669 = case shown="True" w6438 {
                  frame False {
                  }
                  frame True {
                    n3670 = local read "ON L04-2"() -> (w6442:cluster{"amps":dbl, "volts":dbl, "pf":dbl})
                    n3671 = global write "Global display 2.vi" "ON L04-2"(w6442) -> ()
                  }
                }
              }
              frame #8 {
                n3672 = local read "SIG LAB05-1"() -> (w6446:T2)
                n3673 = Unbundle(w6446) -> ("AMPS"=w6445:dbl)  [unwired: 4 out]
                n3674 = Greater?(x=w6445, y=w6444) -> (0:w6443:bool)
                n3675 = case shown="True" w6443 {
                  frame False {
                  }
                  frame True {
                    n3676 = local read "ON L05-1"() -> (w6447:cluster{"amps":dbl, "volts":dbl, "pf":dbl})
                    n3677 = global write "Global display 2.vi" "ON L05-1"(w6447) -> ()
                  }
                }
              }
              frame #9 {
                n3678 = local read "SIG LAB05-2"() -> (w6451:T2)
                n3679 = Unbundle(w6451) -> ("AMPS"=w6450:dbl)  [unwired: 4 out]
                n3680 = Greater?(x=w6450, y=w6449) -> (0:w6448:bool)
                n3681 = case shown="True" w6448 {
                  frame False {
                  }
                  frame True {
                    n3682 = local read "ON L05-2"() -> (w6452:cluster{"amps":dbl, "volts":dbl, "pf":dbl})
                    n3683 = global write "Global display 2.vi" "ON L05-2"(w6452) -> ()
                  }
                }
              }
            }
            n3684 = global write "Global display 3.vi" "TEMP RS 05-2"(w6309) -> ()
            n3685 = global write "Global display 3.vi" "TEMP RS 05-1"(w6310) -> ()
            n3686 = global write "Global display 3.vi" "TEMP RS 03-2"(w6313) -> ()
            n3687 = global write "Global display 3.vi" "TEMP RS 02-1"(w6316) -> ()
            n3688 = global write "Global display 3.vi" "TEMP RS 02-2"(w6315) -> ()
            n3689 = global write "Global display 3.vi" "TEMP RS 04-2"(w6311) -> ()
            n3690 = global write "Global display 3.vi" "TEMP RS 01-2"(w6317) -> ()
            n3691 = global write "Global display 3.vi" "TEMP RS 03-1"(w6314) -> ()
            n3692 = global write "Global display 3.vi" "TEMP RS 04-1"(w6312) -> ()
            n3693 = global write "Global display 3.vi" "TEMP RS 01-1"(w6318) -> ()
            n3694 = global write "Global display 2.vi" "RESULT LAB05-1"(w6354) -> ()
            n3695 = global write "Global display 2.vi" "RESULT LAB01-2"(w6361) -> ()
            n3696 = global write "Global display 2.vi" "RESULT LAB03-2"(w6357) -> ()
            n3697 = global write "Global display 2.vi" "RESULT LAB04-1"(w6356) -> ()
            n3698 = global write "Global display 2.vi" "RESULT LAB04-2"(w6355) -> ()
            n3699 = global write "Global display 2.vi" "RESULT LAB05-2"(w6353) -> ()
            n3700 = global write "Global display 2.vi" "RESULT LAB03-1"(w6358) -> ()
            n3701 = global write "Global display 2.vi" "RESULT LAB01-1"(w6362) -> ()
            n3702 = global write "Global display 2.vi" "RESULT LAB02-1"(w6360) -> ()
            n3703 = global write "Global display 2.vi" "RESULT LAB02-2"(w6359) -> ()
          }
          frame #23 {
            # "simulate values"
            n3704 = global write "Global display 4.vi" "LAB deg C"("LAB deg C") -> ()
          }
          frame #24 {
            # "end main and display program"
            n3705 = stacked-sequence {
              seq-local: [_ w6459 _] -> [_ _ w6466]
              tunnel: w6455 -> [w6456 _ _]
              tunnel: w6454 -> [_ _ w6464]
              frame #0 {
                n3706 = case shown="True" w6456 {
                  frame False {
                  }
                  frame True {
                    n3707 = One Button Dialog(message="Excessive number of USB \nresets done, re-start program.") -> ()  [unwired: 1 in, 1 out]
                  }
                }
              }
              frame #1 {
                # "check for reset error"
                n3708 = local read "DAQ Simulate"() -> (w6458:bool)
                n3709 = case shown="False" w6458 {
                  tunnel: [w6460 FALSE] -> w6459
                  frame False {
                    n3710 = local read "Reset Error"() -> (w6460:bool)
                    n3711 = case shown="True" w6460 {
                      frame False {
                      }
